vi "Install Files.vi"(8 "error in (no error)":errorcluster, 10 "Generated PPL":path, 11 "Builder in":refnum<class "Builder.lvclass">) -> (0 "error out":errorcluster, 2 "PPL Path":path, 3 "Builder out":refnum<class "Builder.lvclass">)   [LabVIEW 2019, in "Builder.lvclass"]
uses:
  Builder.lvclass
  Builder.lvclass/Builder.ctl
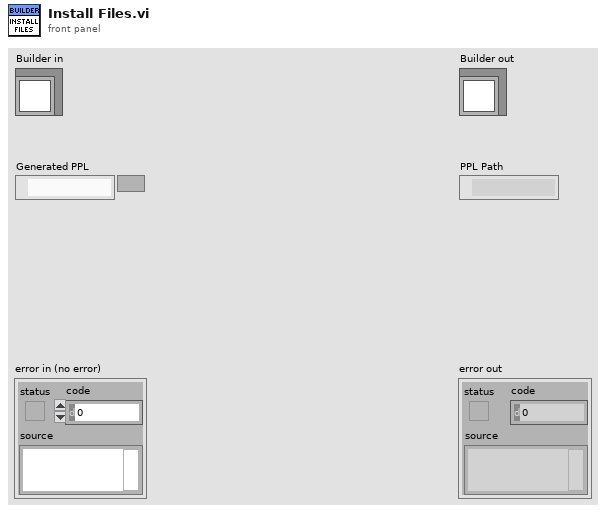
[diagram p1: front panel]
types:
  T1 = typedef "TargetType.ctl" = enum16{"Windows", "cRIO-9045"}
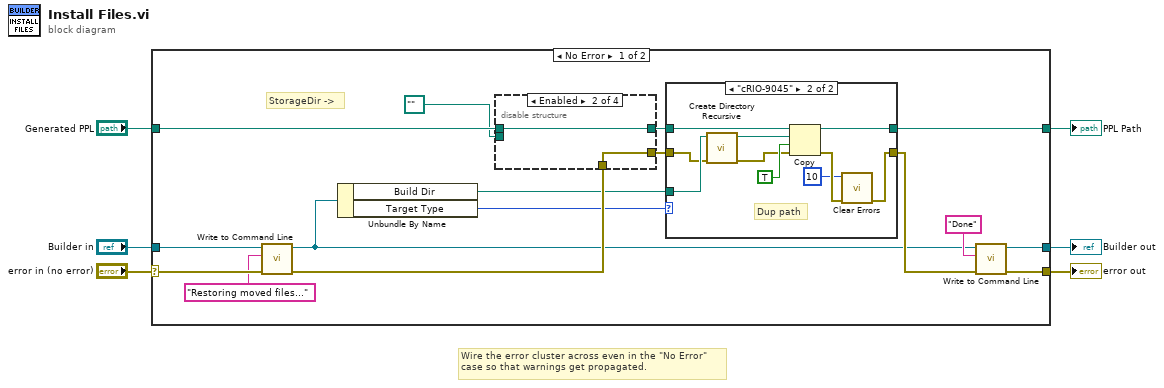
[diagram p0: block diagram]
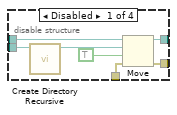
[diagram p2: hidden frame]
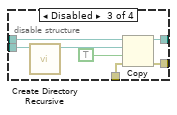
[diagram p3: hidden frame]
diagram:
  # "Wire the error cluster across even in the \"No Error\"\ncase so that warnings get propagated."
  n1 = case shown="No Error" "error in (no error)" {
    selector: "error in (no error)" -> [w20 w55]
    tunnel: [w11 w55] -> w5
    tunnel: [w10 w54] -> w3
    tunnel: "Builder in" -> [w16 w54]
    tunnel: "Generated PPL" -> [w14 w53]
    tunnel: [w7 w53] -> w1
    frame No Error {
      # "StorageDir ->"
      n2 = call "Write to Command Line.vi"("error in (no error)"=w20, "Message"="Restoring moved files...", "Builder in"=w16) -> ("error out"=w21:errorcluster, "Builder out"=w12:refnum<class "Builder.lvclass">)  [unwired: 7 in]
      n3 = Unbundle By Name(w12) -> ("Build Dir"=w8:path, "Target Type"=w13:T1)
      n4 = disable-structure shown="Enabled" {
        disable-tunnel: w21 -> [w29 w30 w38 w39]
        disable-tunnel: [w28 w31 w37 w40] -> w19
        disable-tunnel: [w27 w30 w36 w39] -> w17
        disable-tunnel: w14 -> [w25 w31 w34 w40]
        disable-tunnel: path "" -> [w24 _ w33 _]
        frame Disabled {
          n5 = call <vilib>:"Create Directory Recursive.vi"("directory"=w24) -> ("directory copy"=w23:path)  [unwired: 4 in, 2 out]
          n6 = Move(source path=w25, error in=w29, 9:TRUE ("overwrite (F)"), 10:w23) -> (error out=w27:errorcluster, 3:w28:path)  [unwired: 1 in, 1 out]
        }
        frame Enabled {
        }
        frame Disabled {
          n7 = call <vilib>:"Create Directory Recursive.vi"("directory"=w33) -> ("directory copy"=w32:path)  [unwired: 4 in, 2 out]
          n8 = Copy(8:w38, 9:TRUE ("overwrite (F)"), 10:w32, 11:w34) -> (0:w36:errorcluster, 3:w37:path)  [unwired: 1 in, 1 out]
        }
        frame Disabled {
        }
      }
      n9 = case shown="\"cRIO-9045\"" w13 {
        tunnel: w17 -> [w42 w43]
        tunnel: [w42 w50] -> w18
        tunnel: w19 -> [w41 w51]
        tunnel: w8 -> [_ w45]
        tunnel: [w41 w47] -> w7
        frame "Windows", Default {
        }
        frame "cRIO-9045" {
          # "Dup path"
          n10 = call <vilib>:"Create Directory Recursive.vi"("error in (no error)"=w43, "directory"=w45) -> ("error out"=w44:errorcluster, "directory copy"=w46:path)  [unwired: 3 in, 1 out]
          n11 = Copy(8:w44, 9:TRUE ("overwrite (F)"), 10:w46, 11:w51) -> (0:w52:errorcluster, 3:w47:path)  [unwired: 1 in, 1 out]
          n12 = call <vilib>:"Clear Errors.vi"("error in (no error)"=w52, "specific error code to clear (0: all)"=10) -> ("error out"=w50:errorcluster)  [unwired: 4 in, 1 out]
        }
      }
      n13 = call "Write to Command Line.vi"("error in (no error)"=w18, "Message"="Done", "Builder in"=w12) -> ("error out"=w11:errorcluster, "Builder out"=w10:refnum<class "Builder.lvclass">)  [unwired: 7 in]
    }
    frame Error {
    }
  }
  "error out" <- w5
  "Builder out" <- w3
  "PPL Path" <- w1
